vi "GetGXMLHdr.vi"(8 "error in (no error)":errorcluster, 11 "Channel in":refnum<class "Channel.lvclass">) -> (0 "error out":errorcluster, 2 "ChanHdr":T1, 3 "Channel out":refnum<class "Channel.lvclass">)   [LabVIEW 2012, in "Measurement Channels.lvlib" / "Channel.lvclass"]
uses:
  Channel.lvclass
  ChanProps_TD.ctl
  Channel.lvclass/Channel.ctl
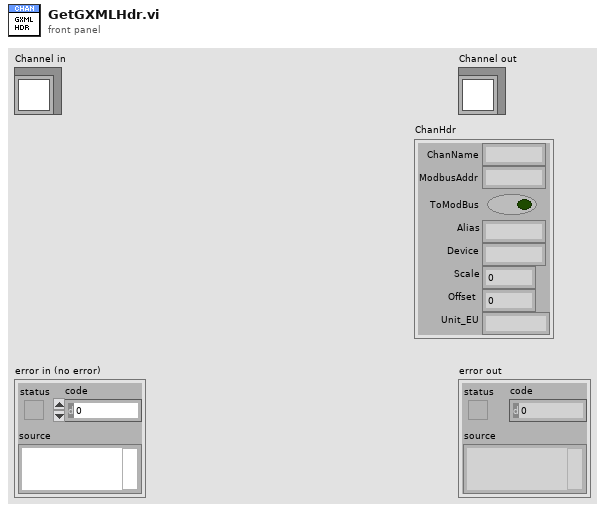
[diagram p1: front panel]
types:
  T1 = typedef "Measurement Channels.lvlib/Channel.lvclass/ChanProps_TD.ctl" = cluster{"ChanName":string, "ModbusAddr":string, "ToModBus":bool, "Alias":string, "Device":string, "Unit_EU":string, "Scale":dbl, "Offset":dbl}
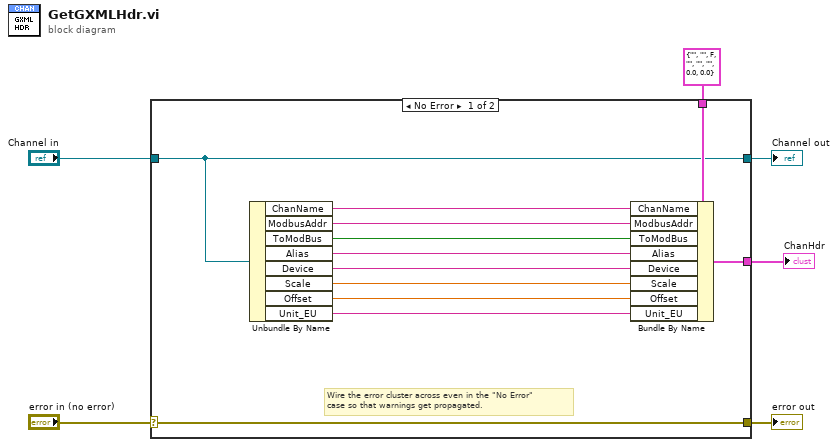
[diagram p0: block diagram]
diagram:
  n1 = case shown="No Error" "error in (no error)" {
    selector: "error in (no error)" -> [w18 w21]
    tunnel: [w18 w21] -> w5
    tunnel: [w15 w20] -> w3
    tunnel: "Channel in" -> [w15 w20]
    tunnel: [w17 w19] -> w2
    tunnel: T1 {"ChanName"="", "ModbusAddr"="", "ToModBus"=FALSE, "Alias"="", "Device"="", "Unit_EU"="", "Scale"=0.0, "Offset"=0.0} ("ChanHdr") -> [w16 w19]
    frame No Error {
      # "Wire the error cluster across even in the \"No Error\"\ncase so that warnings get propagated."
      n2 = Unbundle By Name(w15) -> ("ChanName"=w14:string, "ModbusAddr"=w13:string, "ToModBus"=w12:bool, "Alias"=w11:string, "Device"=w10:string, "Scale"=w9:dbl, "Offset"=w8:dbl, "Unit_EU"=w7:string)
      n3 = Bundle By Name(cluster=w16, "ChanName"=w14, "ModbusAddr"=w13, "ToModBus"=w12, "Alias"=w11, "Device"=w10, "Scale"=w9, "Offset"=w8, "Unit_EU"=w7) -> (w17:T1)
    }
    frame Error {
    }
  }
  "error out" <- w5
  "Channel out" <- w3
  "ChanHdr" <- w2
